vi "battery-reader-dialog.vi"() -> ()   [LabVIEW 2025]
uses:
  <vilib>/addons/_JKI Toolkits/State Machine/_JKI_lib_State_Machine.llb/Select State(s)_err__jki_lib_state_machine.vi
  <vilib>/addons/_JKI Toolkits/State Machine/_JKI_lib_State_Machine.llb/Periodic Trigger__ogtk__JKI-SM__jki_lib_state_machine.vi
  artifacts/battery-prompt/battery-prompt.lvlibp
panel:
  out "DONE":bool
  out "Battery data":T1
  out "Raw content":string
  in  "Restart":bool
  in  "Send request":bool
  in  "Read image":bool
  in  "Exit":bool
  in  "Image selection":enum32{"Camera", "File input"}(tab)
  out "Acquired picture":picture
  in  "Pict Ring":u16(ring)
  out "error out":errorcluster
  in  "error in":errorcluster
  in  "Camera ID":u8
  # "AI-Powered Battery Testing: Prototype Integration of LabVIEW and OpenAI"
  # "1. Select the camera ID and read the image."
  # "2. Use camera input, or select one of the predefined templates."
  # "3. Inspect the data received from the GPT"
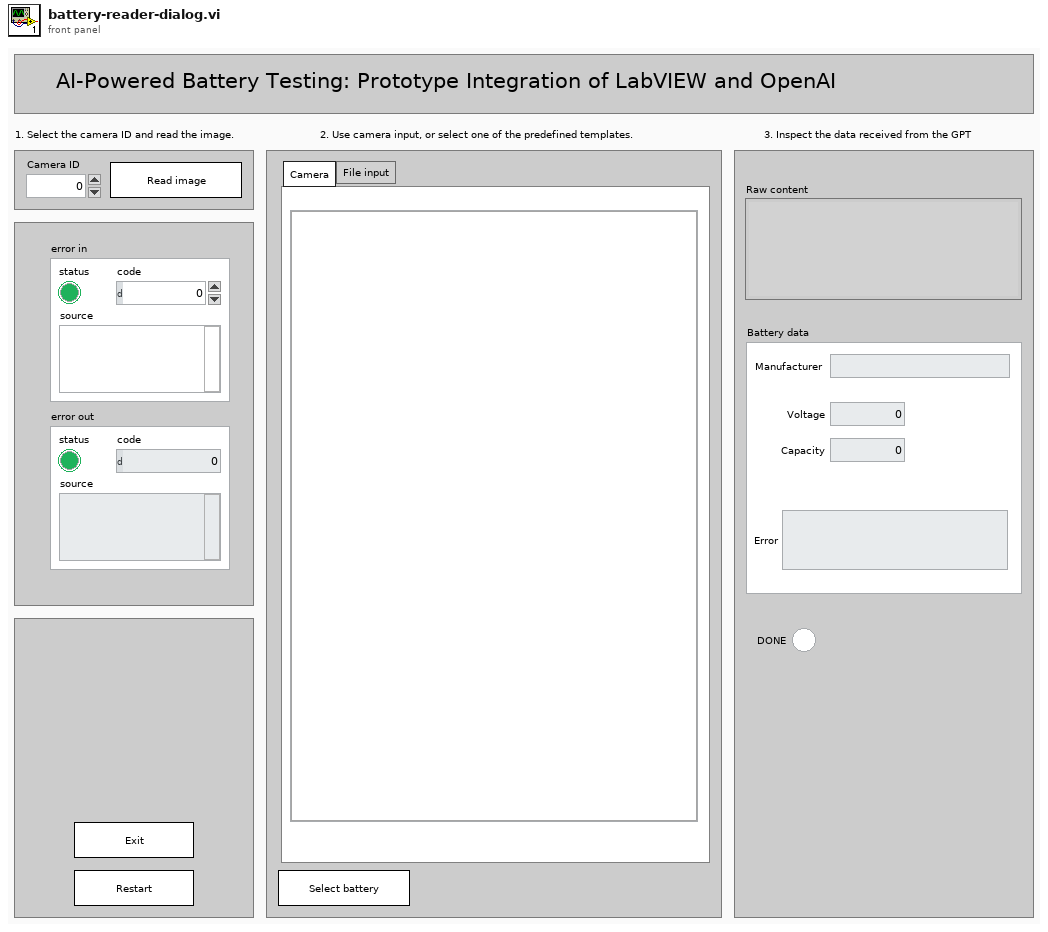
[diagram p1: front panel]
types:
  T1 = cluster{"Manufacturer":string, "Voltage":dbl, "Capacity":u32, "Error":string}
  T2 = enum32{"Invalid", "Standard", "Closed", "Hidden", "Minimized", "Maximized"}
  T3 = enum32{"invalid app kind", "Development System", "Run Time System", "Student Edition", "Embedded LabVIEW", "Evaluation", "Custom"}
  T4 = enum8{"Enabled", "Disabled", "Disabled and Grayed Out"}
  T5 = cluster{"Core":cluster{"Current VI Reference":refnum<vi>, "Close Panel on Exit?":bool}, "Camera ID":u8, "Acquired image":path}
  T6 = cluster{"Current VI Reference":refnum<vi>, "Close Panel on Exit?":bool}
  T7 = typedef "imagedata.ctl" = cluster{"image type":i32, "image depth":i32, "image":u8[], "mask":u8[], "colors":u32[], "Rectangle":cluster{"left":i16, "top":i16, "right":i16, "bottom":i16}}
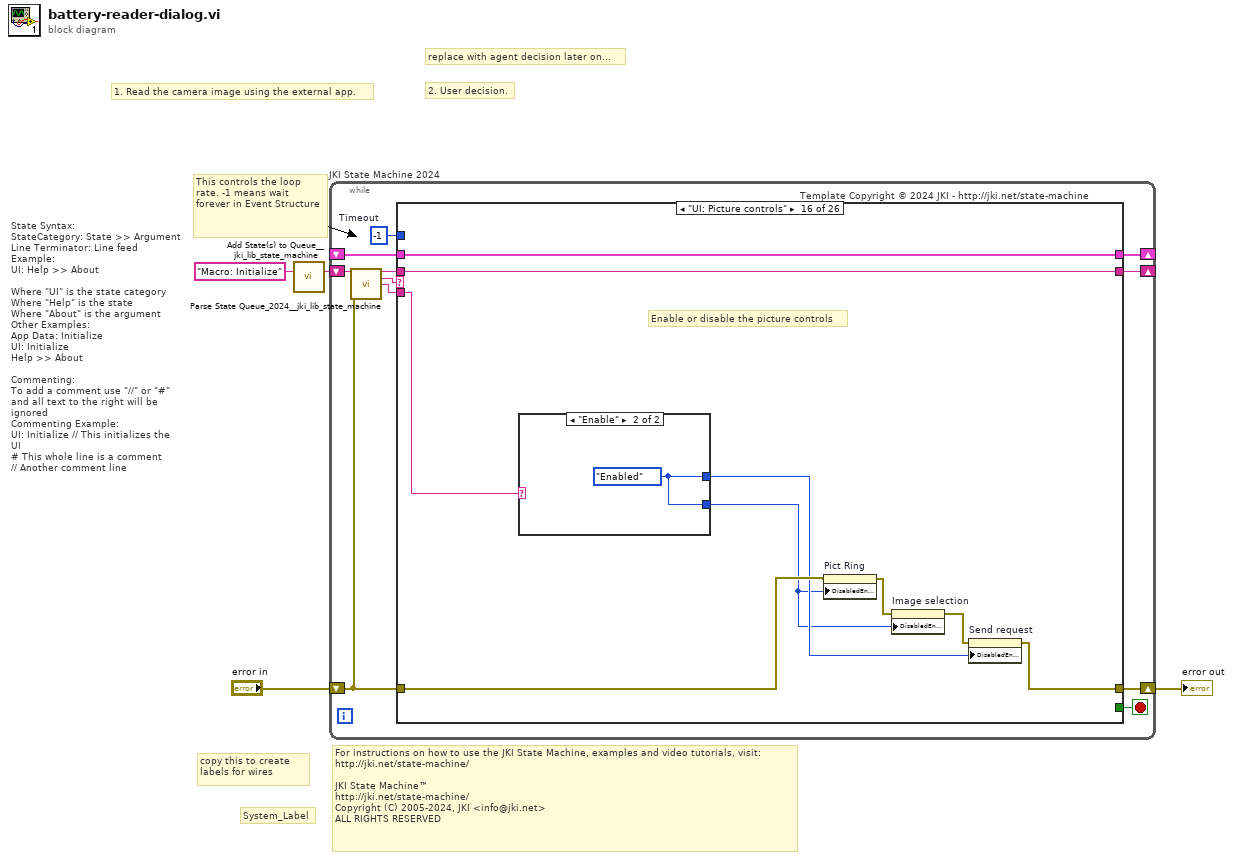
[diagram p0: block diagram]
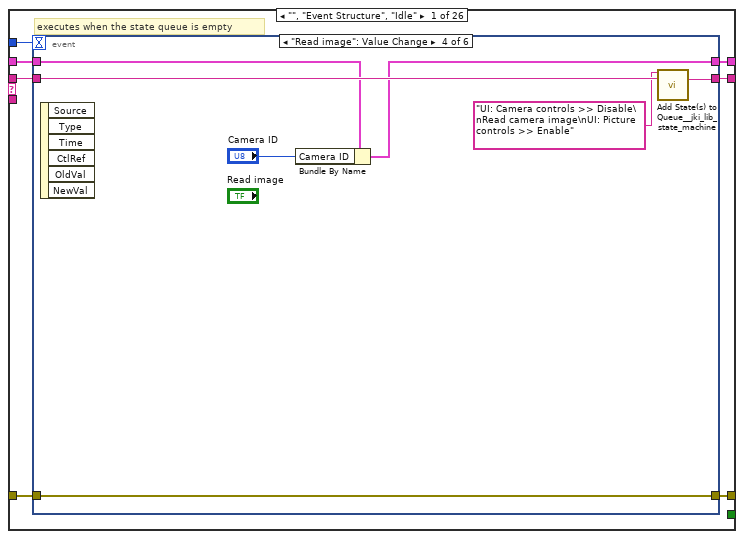
[diagram p2: hidden frame]
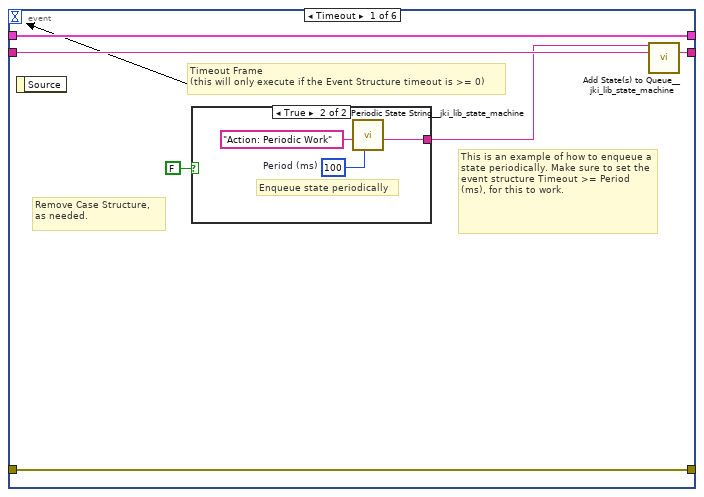
[diagram p3: hidden frame]
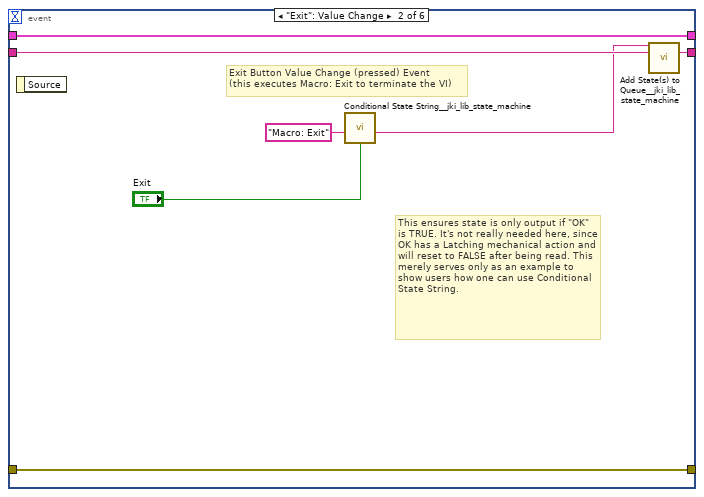
[diagram p5: hidden frame]
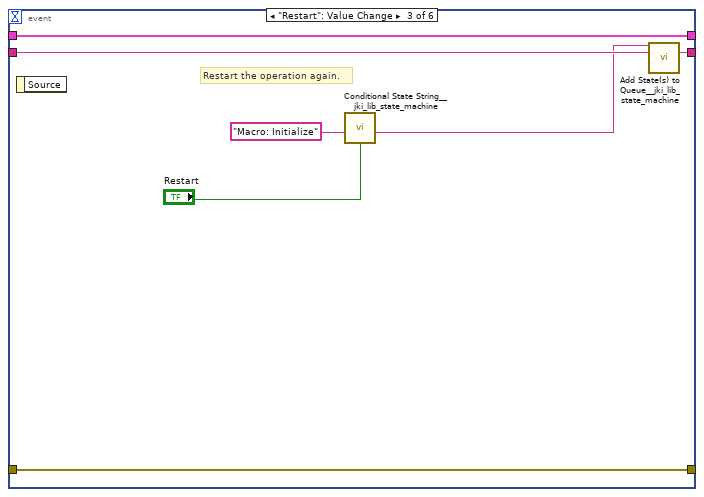
[diagram p6: hidden frame]
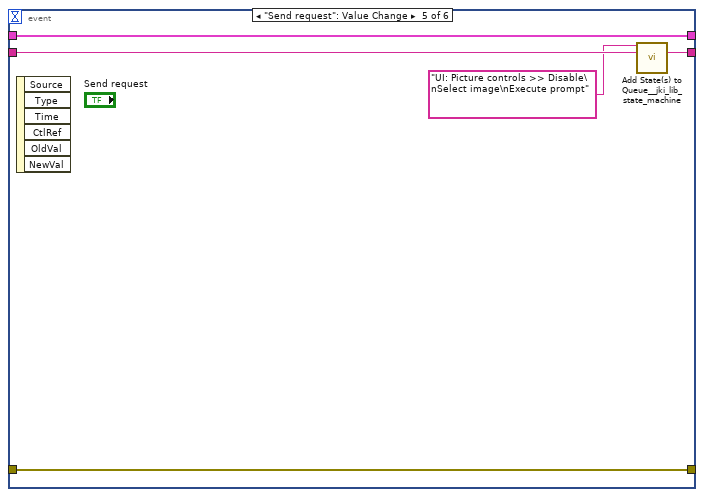
[diagram p7: hidden frame]
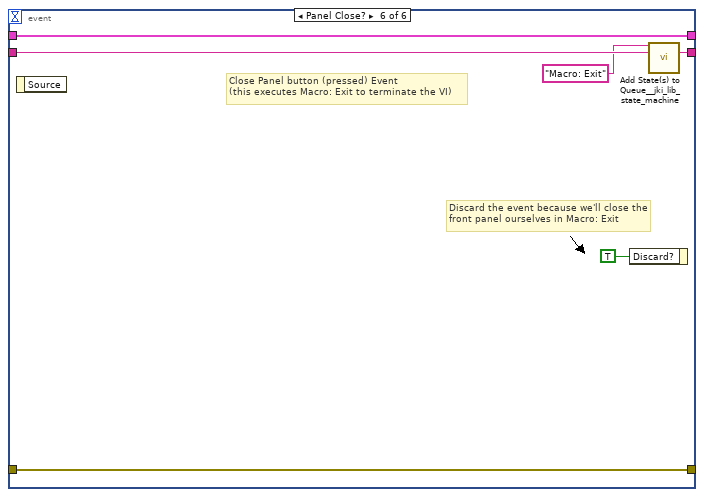
[diagram p8: hidden frame]
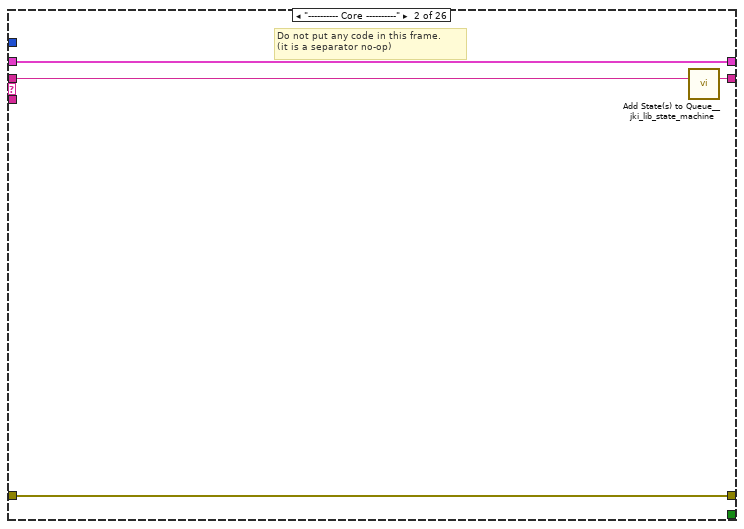
[diagram p9: hidden frame]
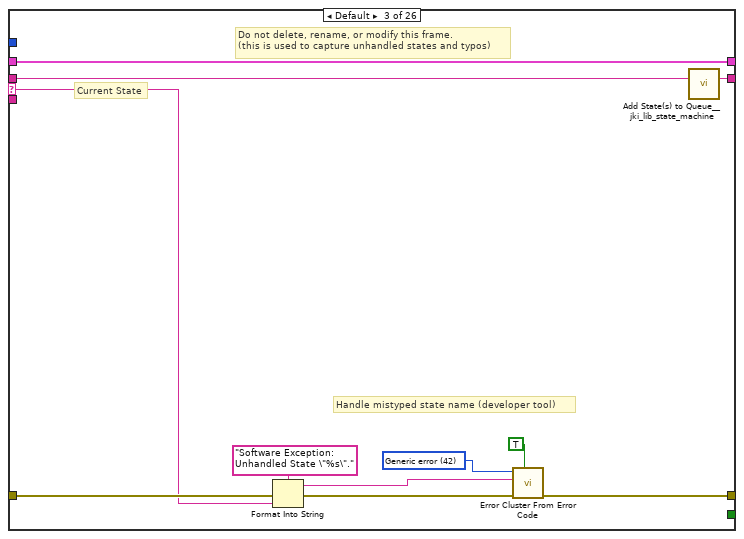
[diagram p10: hidden frame]
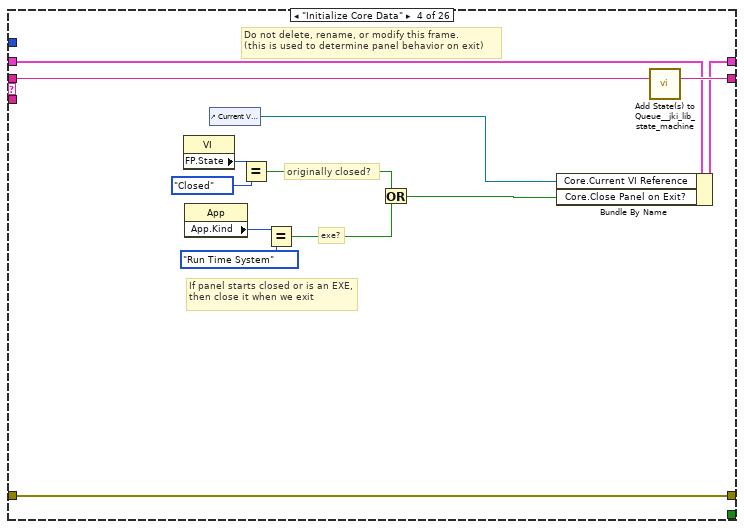
[diagram p11: hidden frame]
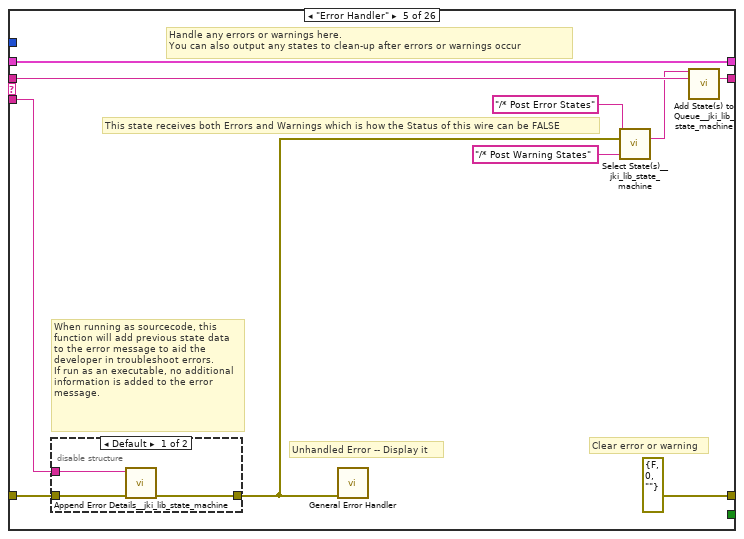
[diagram p12: hidden frame]
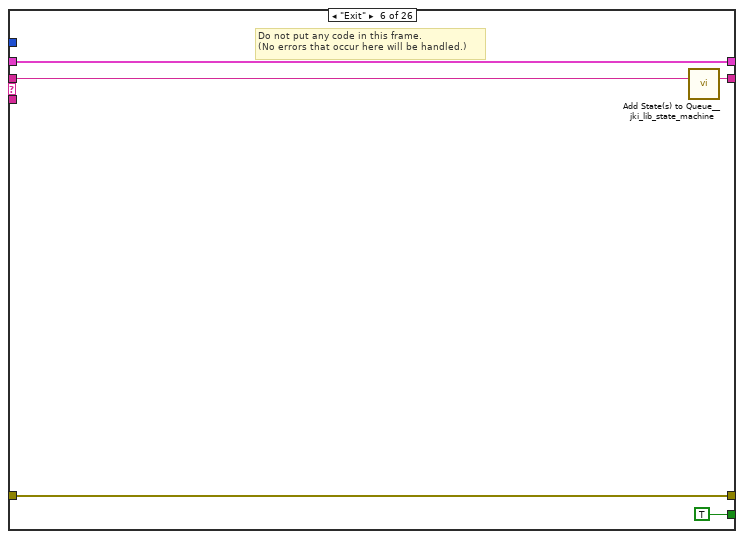
[diagram p14: hidden frame]
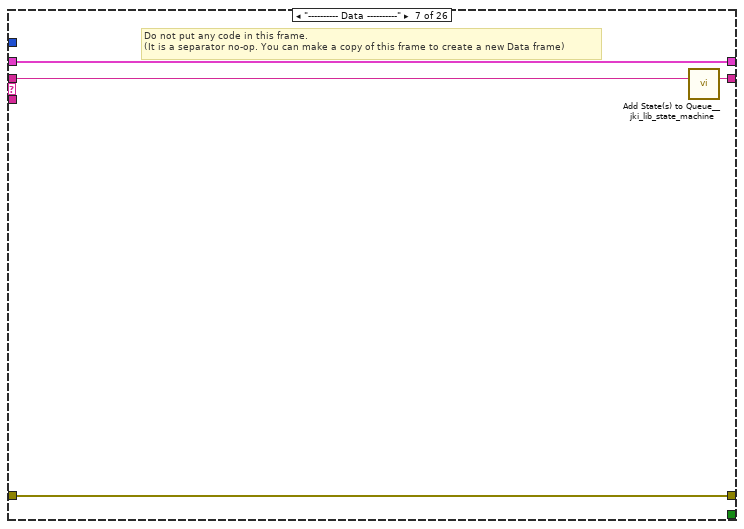
[diagram p15: hidden frame]
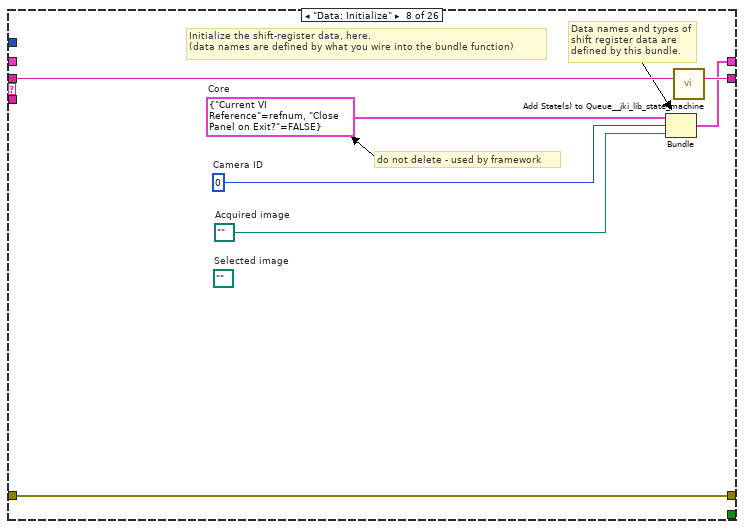
[diagram p16: hidden frame]
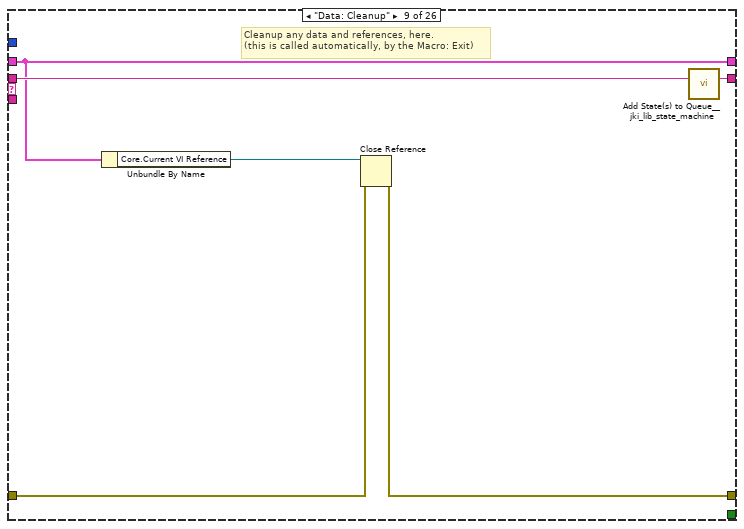
[diagram p17: hidden frame]
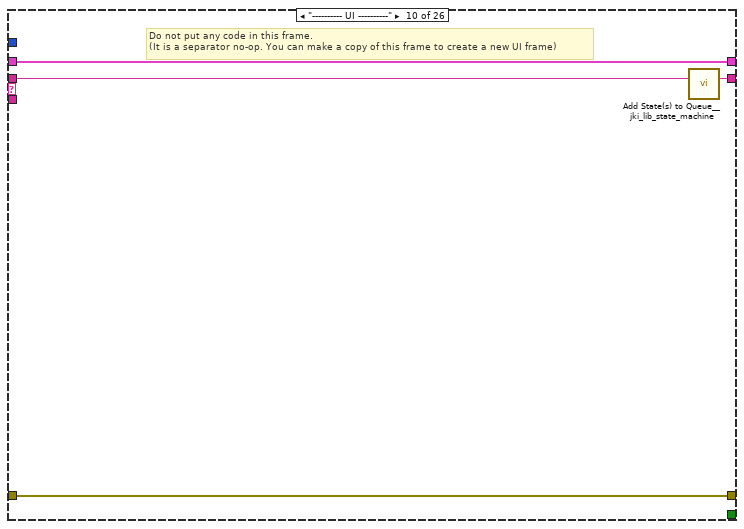
[diagram p18: hidden frame]
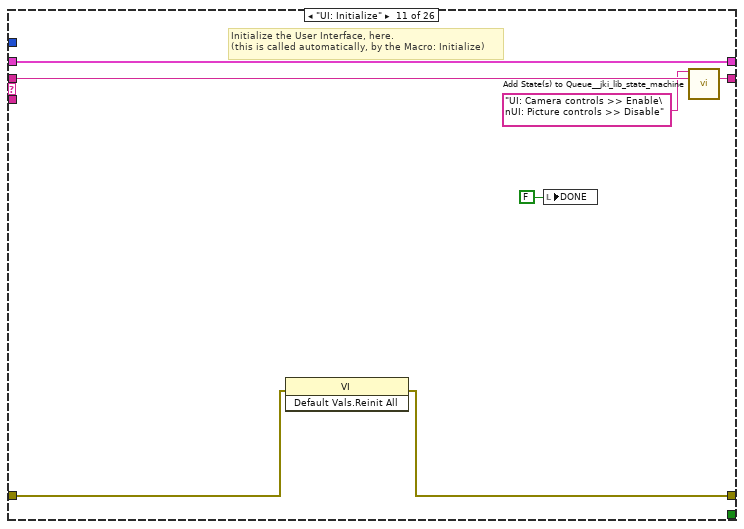
[diagram p19: hidden frame]
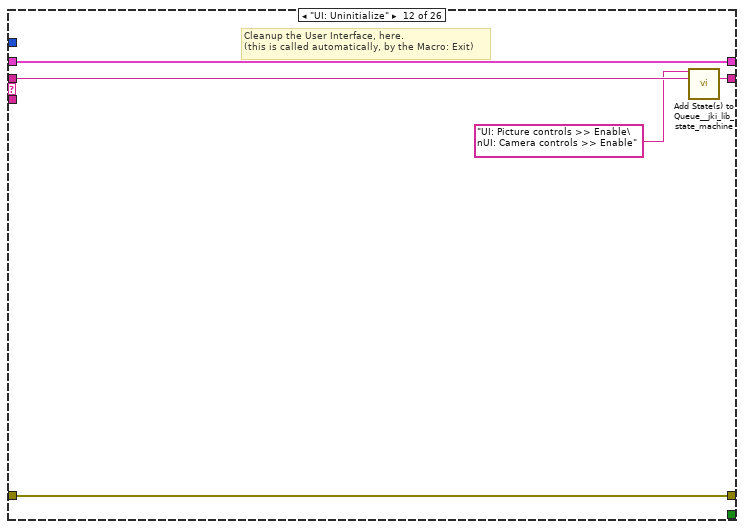
[diagram p20: hidden frame]
diagram:
  # "For instructions on how to use the JKI State Machine, examples and video tutorials, visit:\nhttp://jki.net/state-machine/\n\nJKI State Machine™\nhttp://jki.net/state-machine/\nCopyright (C) 2005-2024, JKI <info@jki.net>\nALL RIGHTS RESERVED"
  # "State Syntax:\nStateCategory: State >> Argument\nLine Terminator: Line feed\nExample:\nUI: Help >> About\n\nWhere \"UI\" is the state category\nWhere \"Help\" is the state\nWhere \"About\" is the argument\nOther Examples:\nApp Data: Initialize\nUI: Initialize\nHelp >> About\n\nCommenting:\nTo add a comment use \"//\" or \"#\" and all text to the right will be ignored\nCommenting Example:\nUI: Initialize // This initializes the UI\n# This whole line is a comment\n// Another comment line"
  # "copy this to create labels for wires"
  # "This controls the loop rate. -1 means wait forever in Event Structure"
  # "System_Label"
  # "replace with agent decision later on..."
  # "2. User decision."
  # "1. Read the camera image using the external app."
  n1 = call <vilib>:"Add State(s) to Queue__jki_lib_state_machine.vi"("State(s) in (\"\")"="Macro: Initialize") -> ("States Out"=w4:string)  [unwired: 14 in]
  n2 = while "JKI State Machine 2024" {
    shift-right: [w8] -> _
    shift-left: _ -> [w7]
    shift-right: [w11] -> w2
    shift-left: "error in" -> [w5]
    shift-right: [w10] -> _
    shift-left: w4 -> [w12]
    stop <- w9 stop-if-true
    w6 = -1  # Timeout
    # "Template Copyright © 2024 JKI - http://jki.net/state-machine"
    n3 = call <vilib>:"Parse State Queue_2024__jki_lib_state_machine.vi"("State Queue"=w12, "Error In (no error)"=w5) -> ("Remaining States"=w14:string, "Current State"=w15:string, "Arguments"=w13:string)  [unwired: 11 in]
    n4 = case shown="\"UI: Picture controls\"" w15 {
      selector: w15 -> [_ _ w68 _ _ _ _ _ _ _ _ _ _ _ _ _ _ _ _ _ _ _ _ _ _ _]
      tunnel: w14 -> [w22 w67 w72 w91 w101 w110 w114 w121 w127 w131 w138 w143 w149 w160 w231 w242 w250 w255 w264 w268 w272 w276 w291 w300 w313 w340]
      tunnel: w13 -> [_ _ _ _ w96 _ _ _ _ _ _ _ w144 w154 w229 w241 _ _ _ _ _ _ _ _ _ w338]
      tunnel: w7 -> [w20 w64 w70 w84 w98 w108 w111 _ w122 w128 w136 w141 w147 w156 w232 w243 w247 w252 w262 w265 w269 w273 w283 w293 w331 w341]
      tunnel: [w19 w65 w74 w88 errorcluster {"status"=FALSE, "code"=0, "source"=""} ("error out") w107 w112 w118 w123 w129 w132 w140 w145 w157 w227 w237 w248 w253 w259 w266 w270 w274 w278 w299 w320 w333] -> w11
      tunnel: w5 -> [w16 w65 w73 w88 w97 w107 w112 w118 w124 w129 w133 w140 w146 w158 w230 w240 w248 w253 w259 w266 w270 w274 w290 w299 w330 w339]
      tunnel: [w21 w66 w71 w90 w100 w109 w113 w120 w126 w130 w137 w142 w148 w159 w231 w242 w249 w254 w263 w267 w271 w275 w291 w300 w314 w340] -> w10
      tunnel: [_ _ _ _ _ TRUE _ _ _ _ _ _ _ _ _ _ _ _ _ _ _ _ _ _ _ _] -> w9
      tunnel: [w18 w64 w70 w89 w98 w108 w111 w119 w122 w128 w136 w141 w147 w156 w232 w243 w247 w252 w262 w265 w269 w273 w282 w292 w331 w341] -> w8
      tunnel: w6 -> [w17 _ _ _ _ _ _ _ _ _ _ _ _ _ _ _ _ _ _ _ _ _ _ _ _ _]
      frame "", "Event Structure", "Idle" {
        # "executes when the state queue is empty"
        n5 = event shown="[3] \"Read image\": Value Change" {
          selector: _ -> [_ _ _ _ _ _]
          dyn-events: _ -> [_ _ _ _ _ _]
          timeout: w17 -> [_ _ _ _ _ _]
          tunnel: w22 -> [w28 w38 w45 w52 w55 w63]
          tunnel: [w27 w37 w44 w51 w56 w62] -> w21
          tunnel: w20 -> [w25 w35 w42 w48 w57 w60]
          tunnel: [w26 w36 w43 w49 w53 w61] -> w19
          tunnel: w16 -> [w26 w36 w43 w49 w53 w61]
          tunnel: [w25 w35 w42 w46 w57 w60] -> w18
          event Timeout {
            # "Remove Case Structure, as needed."
            # "This is an example of how to enqueue a state periodically. Make sure to set the event structure Timeout >= Period (ms), for this to work."
            # "Timeout Frame\n(this will only execute if the Event Structure timeout is >= 0)"
            n6 = event-data() -> ()  [unwired: 1 in, 1 out]
            n7 = case shown="True" FALSE {
              tunnel: [_ w31] -> w24
              frame False {
              }
              frame True {
                w29 = u32 100  # Period (ms)
                # "Enqueue state periodically"
                n8 = call <vilib>:"Periodic State String__jki_lib_state_machine.vi"("Period (ms)"=w29, "State"="Action: Periodic Work") -> ("State Out"=w31:string)  [unwired: 9 in]
              }
            }
            n9 = call <vilib>:"Add State(s) to Queue__jki_lib_state_machine.vi"("State(s) in Front (\"\")"=w24, "State(s) in (\"\")"=w28) -> ("States Out"=w27:string)  [unwired: 13 in]
          }
          event "Exit": Value Change {
            # "This ensures state is only output if \"OK\" is TRUE. It's not really needed here, since OK has a Latching mechanical action and will reset to FALSE after being read. This merely serves only as an example to show users how one can use Conditional State String."
            # "Exit Button Value Change (pressed) Event\n(this executes Macro: Exit to terminate the VI)"
            n10 = event-data() -> ()  [unwired: 1 in, 1 out]
            n11 = call <vilib>:"Conditional State String__jki_lib_state_machine.vi"("Do State(s)?"="Exit", "State"="Macro: Exit") -> ("State Out"=w32:string)  [unwired: 7 in]
            n12 = call <vilib>:"Add State(s) to Queue__jki_lib_state_machine.vi"("State(s) in Front (\"\")"=w32, "State(s) in (\"\")"=w38) -> ("States Out"=w37:string)  [unwired: 13 in]
          }
          event "Restart": Value Change {
            # "Restart the operation again."
            n13 = event-data() -> ()  [unwired: 1 in, 1 out]
            n14 = call <vilib>:"Conditional State String__jki_lib_state_machine.vi"("Do State(s)?"="Restart", "State"="Macro: Initialize") -> ("State Out"=w40:string)  [unwired: 7 in]
            n15 = call <vilib>:"Add State(s) to Queue__jki_lib_state_machine.vi"("State(s) in Front (\"\")"=w40, "State(s) in (\"\")"=w45) -> ("States Out"=w44:string)  [unwired: 13 in]
          }
          event "Read image": Value Change {
            n16 = event-data() -> ()  [unwired: 1 in, 6 out]
            n17 = Bundle By Name(cluster=w48, "Camera ID"="Camera ID") -> (w46:T5)
            n18 = call <vilib>:"Add State(s) to Queue__jki_lib_state_machine.vi"("State(s) in Front (\"\")"="UI: Camera controls >> Disable\nRead camera image\nUI: Picture controls >> Enable" ("State(s) in Front (\"\")"), "State(s) in (\"\")"=w52) -> ("States Out"=w51:string)  [unwired: 13 in]
          }
          event "Send request": Value Change {
            n19 = event-data() -> ()  [unwired: 1 in, 6 out]
            n20 = call <vilib>:"Add State(s) to Queue__jki_lib_state_machine.vi"("State(s) in Front (\"\")"="UI: Picture controls >> Disable\nSelect image\nExecute prompt" ("State(s) in Front (\"\")"), "State(s) in (\"\")"=w55) -> ("States Out"=w56:string)  [unwired: 13 in]
          }
          event Panel Close? {
            # "Discard the event because we'll close the front panel ourselves in Macro: Exit"
            # "Close Panel button (pressed) Event\n(this executes Macro: Exit to terminate the VI)"
            n21 = event-data() -> ()  [unwired: 1 in, 1 out]
            n22 = event-data("Discard?"=TRUE) -> ()  [unwired: 1 in, 1 out]
            n23 = call <vilib>:"Add State(s) to Queue__jki_lib_state_machine.vi"("State(s) in Front (\"\")"="Macro: Exit", "State(s) in (\"\")"=w63) -> ("States Out"=w62:string)  [unwired: 13 in]
          }
        }
      }
      frame "---------- Core ----------" {
        # "Do not put any code in this frame.\n(it is a separator no-op)"
        n24 = call <vilib>:"Add State(s) to Queue__jki_lib_state_machine.vi"("State(s) in (\"\")"=w67) -> ("States Out"=w66:string)  [unwired: 14 in]
      }
      frame Default {
        w77 = 42 items=["No error", "Argument error", "Memory is full", "Out of zone", "End of file", "File already open", "Generic file I/O error", "File not found", "File permission error", "Disk is full", "Duplicate path", "Too many files open", "System feature not enabled", "Resource file not found", "Cannot add resource", "Resource not found", "Image not found", "Image memory error", "Pen does not exist", "Config type invalid", "Config token not found", "Config parse error", "Config memory error", "Bad external code format", "Bad external code offset", "External code not present", "Null window", "Destroy window error", "Null menu", "Print aborted", "Bad print record", "Print driver error", "Windows error during printing", "Memory error during printing", "Print dialog error", "Generic print error", "Invalid device refnum", "Device not found", "Device parameter error", "Device unit error", "Cannot open device", "Device call aborted", "Generic error", "Cancelled by user", "Object ID too low", "Object ID too high", "Object not in heap", "Unknown heap", "Unknown object (invalid DefProc)", "Unknown object (DefProc not in table)", "Message out of range", "Invalid (null) method", "Unknown message", "Manager call not supported", "Bad address", "Network operation in progress", "Network operation timed out", "Connection is busy", "Network attribute not supported", "Network error", "Address in use", "System out of memory", "Connection aborted", "Connection refused", "Not connected", "Already connected", "Connection closed", "Initialization error (interapplication manager)", "Bad occurrence", "Wait on unbound occurrence handler", "Occurrence queue overflow", "Datalog type conflict", "Unused", "Unrecognized type (interapplication manager)", "Memory corrupt", "Failed to make temporary DLL", "Old CIN version", "Drag socket not found", "Failed to load drop-object", "Failed to register OLE object", "Failed to release OLE object", "Format specifier type mismatch", "Unknown format specifier", "Too few format specifiers", "Too many format specifiers", "Scan failed", "Newer CIN version", "Error converting to variant", "Runtime menu error", "Password tampered", "Variant attribute not found", "Incompatible variant data type", "Event data is not available", "Event Store is not present", "Occurrence is not found", "Event Queue is not created", "Event info is not available", "Refnum passed is NULL", "Error retrieving Class GUID", "Error retrieving CoClass GUID", "Error retrieving TypeLib GUID.", "Bad built application magic bytes.", "Specific driver is different from the specific driver associated with the Logical Name.", "There is no session opened to the class driver.", "Max Error", "MAX - Error with config objects", "MAX - Error loading configuration", "MAX - Group not supported"]
        # "Current State"
        # "Do not delete, rename, or modify this frame.\n(this is used to capture unhandled states and typos)"
        # "Handle mistyped state name (developer tool)"
        n25 = Format Into String(format string="Software Exception: Unhandled State \"%s\"." ("message"), error in=w73, w68) -> (resulting string=w76:string, error out=w75:errorcluster)  [unwired: 1 in]
        n26 = call <vilib>:"Error Cluster From Error Code.vi"("show call chain? (False)"=TRUE, "error in (no error)"=w75, "error message (\"\")"=w76, "error code (0)"=w77) -> ("error out"=w74:errorcluster)  [unwired: 5 in]
        n27 = call <vilib>:"Add State(s) to Queue__jki_lib_state_machine.vi"("State(s) in (\"\")"=w72) -> ("States Out"=w71:string)  [unwired: 14 in]
      }
      frame "Initialize Core Data" {
        # "Do not delete, rename, or modify this frame.\n(this is used to determine panel behavior on exit)"
        # "originally closed?"
        # "exe?"
        # "If panel starts closed or is an EXE, then close it when we exit"
        n28 = property class="VI"() -> ("FP.State"=w81:T2)  [unwired: 2 in, 2 out]
        n29 = property class="App"() -> ("App.Kind"=w87:T3)  [unwired: 2 in, 2 out]
        n30 = control-ref of="Current VI Reference"() -> (w82:refnum<vi>)
        n31 = Equal?(x=w81, y=T2."Closed" ("Front Panel Window:State")) -> (x = y?=w79:bool)
        n32 = Equal?(x=w87, y=T3."Run Time System" ("Application:Kind")) -> (x = y?=w85:bool)
        n33 = Or(x=w79, y=w85) -> (x .or. y?=w83:bool)
        n34 = Bundle By Name(cluster=w84, "Core.Current VI Reference"=w82, "Core.Close Panel on Exit?"=w83) -> (w89:T5)
        n35 = call <vilib>:"Add State(s) to Queue__jki_lib_state_machine.vi"("State(s) in (\"\")"=w91) -> ("States Out"=w90:string)  [unwired: 14 in]
      }
      frame "Error Handler" {
        # "When running as sourcecode, this function will add previous state data to the error message to aid the developer in troubleshoot errors.\nIf run as an executable, no additional information is added to the error message."
        # "This state receives both Errors and Warnings which is how the Status of this wire can be FALSE"
        # "Unhandled Error -- Display it"
        # "Handle any errors or warnings here.\nYou can also output any states to clean-up after errors or warnings occur"
        # "Clear error or warning"
        n36 = disable-structure shown="Default" {
          disable-tunnel: w97 -> [w104 w105]
          disable-tunnel: w96 -> [w103 _]
          disable-tunnel: [w102 w105] -> w95
          frame condition #0 (active) {
            n37 = call <vilib>:"Append Error Details__jki_lib_state_machine.vi"("error in (no error)"=w104, "Previous State and Argument(s)"=w103) -> ("error out"=w102:errorcluster)  [unwired: 9 in]
          }
          frame condition #1 {
          }
        }
        n38 = call <vilib>:"General Error Handler.vi"("error in (no error)"=w95) -> ()  [unwired: 10 in, 5 out]
        n39 = call-poly <vilib>:"Select State(s)__jki_lib_state_machine.vi"("State(s) if True (\"\")"="/* Post Error States", "Select"=w95, "State(s) if False (\"\")"="/* Post Warning States") -> ("States Out"=w93:string)  [unwired: 12 in]
        n40 = call <vilib>:"Add State(s) to Queue__jki_lib_state_machine.vi"("State(s) in Front (\"\")"=w93, "State(s) in (\"\")"=w101) -> ("States Out"=w100:string)  [unwired: 13 in]
      }
      frame "Exit" {
        # "Do not put any code in this frame.\n(No errors that occur here will be handled.)"
        n41 = call <vilib>:"Add State(s) to Queue__jki_lib_state_machine.vi"("State(s) in (\"\")"=w110) -> ("States Out"=w109:string)  [unwired: 14 in]
      }
      frame "---------- Data ----------" {
        # "Do not put any code in this frame.\n(It is a separator no-op. You can make a copy of this frame to create a new Data frame)"
        n42 = call <vilib>:"Add State(s) to Queue__jki_lib_state_machine.vi"("State(s) in (\"\")"=w114) -> ("States Out"=w113:string)  [unwired: 14 in]
      }
      frame "Data: Initialize" {
        (unwired) path ""  # Selected image
        w115 = path ""  # Acquired image
        w116 = u8 0  # Camera ID
        w117 = T6 {"Current VI Reference"=refnum, "Close Panel on Exit?"=FALSE}  # Core
        # "do not delete - used by framework"
        # "Data names and types of shift register data are defined by this bundle."
        # "Initialize the shift-register data, here.\n(data names are defined by what you wire into the bundle function)"
        n43 = Bundle("Core"=w117, "Camera ID"=w116, "Acquired image"=w115) -> (w119:T5)  [unwired: 1 in]
        n44 = call <vilib>:"Add State(s) to Queue__jki_lib_state_machine.vi"("State(s) in (\"\")"=w121) -> ("States Out"=w120:string)  [unwired: 14 in]
      }
      frame "Data: Cleanup" {
        # "Cleanup any data and references, here.\n(this is called automatically, by the Macro: Exit)"
        n45 = Unbundle By Name(w122) -> ("Core.Current VI Reference"=w125:refnum<vi>)
        n46 = Close Reference(reference=w125, error in (no error)=w124) -> (error out=w123:errorcluster)
        n47 = call <vilib>:"Add State(s) to Queue__jki_lib_state_machine.vi"("State(s) in (\"\")"=w127) -> ("States Out"=w126:string)  [unwired: 14 in]
      }
      frame "---------- UI ----------" {
        # "Do not put any code in this frame.\n(It is a separator no-op. You can make a copy of this frame to create a new UI frame)"
        n48 = call <vilib>:"Add State(s) to Queue__jki_lib_state_machine.vi"("State(s) in (\"\")"=w131) -> ("States Out"=w130:string)  [unwired: 14 in]
      }
      frame "UI: Initialize" {
        # "Initialize the User Interface, here.\n(this is called automatically, by the Macro: Initialize)"
        n49 = invoke class="VI" method="Default Vals.Reinit All"(error in=w133) -> (error out=w132:errorcluster)  [unwired: 2 in, 2 out]
        n50 = local write "DONE"(FALSE ("DONE")) -> ()
        n51 = call <vilib>:"Add State(s) to Queue__jki_lib_state_machine.vi"("State(s) in Front (\"\")"="UI: Camera controls >> Enable\nUI: Picture controls >> Disable" ("State(s) in Front (\"\")"), "State(s) in (\"\")"=w138) -> ("States Out"=w137:string)  [unwired: 13 in]
      }
      frame "UI: Uninitialize" {
        # "Cleanup the User Interface, here.\n(this is called automatically, by the Macro: Exit)"
        n52 = call <vilib>:"Add State(s) to Queue__jki_lib_state_machine.vi"("State(s) in Front (\"\")"="UI: Picture controls >> Enable\nUI: Camera controls >> Enable" ("State(s) in Front (\"\")"), "State(s) in (\"\")"=w143) -> ("States Out"=w142:string)  [unwired: 13 in]
      }
      frame "UI: Cursor Set" {
        # "Argument"
        # "Set and Unset Cursor Busy.\n(Usage: \"UI: Cursor Set >> Busy|Idle\")"
        n53 = case shown="\"Idle\", Default" w144 {
          tunnel: w146 -> [w151 w153]
          tunnel: [w150 w152] -> w145
          frame "Idle", Default {
            n54 = call <vilib>:"Unset Busy.vi"("error in (no error)"=w151) -> ("error out"=w150:errorcluster)  [unwired: 10 in]
          }
          frame "Busy" {
            n55 = call <vilib>:"Set Busy.vi"("error in (no error)"=w153) -> ("error out"=w152:errorcluster)  [unwired: 9 in, 1 out]
          }
        }
        n56 = call <vilib>:"Add State(s) to Queue__jki_lib_state_machine.vi"("State(s) in (\"\")"=w149) -> ("States Out"=w148:string)  [unwired: 14 in]
      }
      frame "UI: Front Panel State" {
        # "Argument"
        # "Set Front Panel Open or Closed\n(Usage: \"UI: Front Panel State >> Open|Close\")"
        n57 = Unbundle By Name(w156) -> ("Core.Current VI Reference"=w155:refnum<vi>)
        n58 = case shown="\"Close\", \"Closed\"" w154 {
          tunnel: w158 -> [w166 w181 w192 w205 w218]
          tunnel: [w168 w182 w194 w207 w220] -> w157
          tunnel: w155 -> [w167 w179 w193 w206 w219]
          frame "Open", "Standard", Default {
            w161 = T2."Standard" ("State")
            n59 = property class="VI"(reference=w167, error in=w166) -> (reference out=w164:refnum<vi>, error out=w165:errorcluster, "FP.State"=w163:T2)
            n60 = Not Equal?(x=w163, y=w161) -> (x != y?=w162:bool)
            n61 = case shown="True" w162 {
              tunnel: [w172 w174] -> w168
              tunnel: w165 -> [w171 w174]
              tunnel: w164 -> [w170 _]
              tunnel: w161 -> [w169 _]
              frame True {
                n62 = invoke class="VI" method="FP.Open"(reference=w170, error in=w171, "Activate"=TRUE, "State"=w169) -> (error out=w172:errorcluster)  [unwired: 1 in, 4 out]
              }
              frame False {
              }
            }
          }
          frame "Close", "Closed" {
            n63 = property class="VI"(reference=w179, error in=w181) -> (reference out=w178:refnum<vi>, error out=w180:errorcluster, "FP.State"=w176:T2)
            n64 = Not Equal?(x=w176, y=T2."Closed" ("Front Panel Window:State")) -> (x != y?=w175:bool)
            n65 = case shown="True" w175 {
              tunnel: [w183 w186] -> w182
              tunnel: w180 -> [w183 w185]
              tunnel: w178 -> [_ w184]
              frame False {
              }
              frame True {
                n66 = invoke class="VI" method="FP.Close"(reference=w184, error in=w185) -> (error out=w186:errorcluster)  [unwired: 1 in, 2 out]
              }
            }
          }
          frame "Hidden", "Hide" {
            w187 = T2."Hidden" ("State")
            n67 = property class="VI"(reference=w193, error in=w192) -> (reference out=w190:refnum<vi>, error out=w191:errorcluster, "FP.State"=w189:T2)
            n68 = Not Equal?(x=w189, y=w187) -> (x != y?=w188:bool)
            n69 = case shown="True" w188 {
              tunnel: [w198 w199] -> w194
              tunnel: w191 -> [w197 w199]
              tunnel: w190 -> [w196 _]
              tunnel: w187 -> [w195 _]
              frame True {
                n70 = invoke class="VI" method="FP.Open"(reference=w196, error in=w197, "State"=w195) -> (error out=w198:errorcluster)  [unwired: 2 in, 4 out]
              }
              frame False {
              }
            }
          }
          frame "Minimize", "Minimized" {
            w200 = T2."Minimized" ("State")
            n71 = property class="VI"(reference=w206, error in=w205) -> (reference out=w203:refnum<vi>, error out=w204:errorcluster, "FP.State"=w202:T2)
            n72 = Not Equal?(x=w202, y=w200) -> (x != y?=w201:bool)
            n73 = case shown="True" w201 {
              tunnel: [w211 w212] -> w207
              tunnel: w204 -> [w210 w212]
              tunnel: w203 -> [w209 _]
              tunnel: w200 -> [w208 _]
              frame True {
                n74 = invoke class="VI" method="FP.Open"(reference=w209, error in=w210, "State"=w208) -> (error out=w211:errorcluster)  [unwired: 2 in, 4 out]
              }
              frame False {
              }
            }
          }
          frame "Maximize", "Maximized" {
            w213 = T2."Maximized" ("State")
            n75 = property class="VI"(reference=w219, error in=w218) -> (reference out=w216:refnum<vi>, error out=w217:errorcluster, "FP.State"=w215:T2)
            n76 = Not Equal?(x=w215, y=w213) -> (x != y?=w214:bool)
            n77 = case shown="True" w214 {
              tunnel: [w224 w225] -> w220
              tunnel: w217 -> [w223 w225]
              tunnel: w216 -> [w222 _]
              tunnel: w213 -> [w221 _]
              frame True {
                n78 = invoke class="VI" method="FP.Open"(reference=w222, error in=w223, "State"=w221) -> (error out=w224:errorcluster)  [unwired: 2 in, 4 out]
              }
              frame False {
              }
            }
          }
        }
        n79 = call <vilib>:"Add State(s) to Queue__jki_lib_state_machine.vi"("State(s) in (\"\")"=w160) -> ("States Out"=w159:string)  [unwired: 14 in]
      }
      frame "UI: Camera controls" {
        # "Enable or disable the camera controls"
        n80 = case shown="\"Enable\"" w229 {
          tunnel: [T4."Disabled and Grayed Out" ("Disabled") T4."Enabled" ("Disabled")] -> w226
          frame "Disable", Default {
          }
          frame "Enable" {
          }
        }
        n81 = property on="Camera ID" class="DigNum (strict)"(error in=w230, "DisabledEnum"=w226) -> (error out=w228:errorcluster)  [unwired: 1 in, 1 out]
        n82 = property on="Read image" class="Bool"(error in=w228, "DisabledEnum"=w226) -> (error out=w227:errorcluster)  [unwired: 1 in, 1 out]
      }
      frame "UI: Picture controls" {
        # "Enable or disable the picture controls"
        n83 = case shown="\"Enable\"" w241 {
          tunnel: [T4."Disabled and Grayed Out" ("Disabled") w246] -> w236
          tunnel: [T4."Disabled" ("Disabled") w246] -> w235
          frame "Disable", Default {
          }
          frame "Enable" {
            w246 = T4."Enabled" ("Disabled")
          }
        }
        n84 = property on="Pict Ring" class="Ring (strict)"(error in=w240, "DisabledEnum"=w235) -> (error out=w239:errorcluster)  [unwired: 1 in, 1 out]
        n85 = property on="Image selection" class="TabCtl (strict)"(error in=w239, "DisabledEnum"=w235) -> (error out=w238:errorcluster)  [unwired: 1 in, 1 out]
        n86 = property on="Send request" class="Bool"(error in=w238, "DisabledEnum"=w236) -> (error out=w237:errorcluster)  [unwired: 1 in, 1 out]
      }
      frame "---------- Macro ----------" {
        # "Do not put any code in this frame.\n(It is a separator no-op. You can make a copy of this frame to create a new Macro frame)"
        n87 = call <vilib>:"Add State(s) to Queue__jki_lib_state_machine.vi"("State(s) in (\"\")"=w250) -> ("States Out"=w249:string)  [unwired: 14 in]
      }
      frame "Macro: Initialize" {
        w251 = "Data: Initialize\nInitialize Core Data\nUI: Initialize\nUI: Front Panel State >> Open"  # Data: Initialize Initialize Core Data UI: Initialize UI: Front Panel State >> Open
        # "Initialization Macro\n(This is called once, when the VI starts)"
        n88 = call <vilib>:"Add State(s) to Queue__jki_lib_state_machine.vi"("State(s) in Front (\"\")"=w251, "State(s) in (\"\")"=w255) -> ("States Out"=w254:string)  [unwired: 13 in]
      }
      frame "Macro: Exit" {
        # "Exit Macro\n(This is called once, when the VI exits)"
        n89 = Unbundle By Name(w262) -> ("Core.Close Panel on Exit?"=w257:bool)
        n90 = call <vilib>:"Conditional State String__jki_lib_state_machine.vi"("Do State(s)?"=w257, "State"="UI: Front Panel State >> Close") -> ("State Out"=w256:string)  [unwired: 7 in]
        n91 = call <vilib>:"Add State(s) to Queue__jki_lib_state_machine.vi"("State(s) in (\"\")"=w256, "State(s) at Back (\"\")"="UI: Uninitialize\nData: Cleanup\nExit") -> ("States Out"=w260:string)  [unwired: 13 in]
        n92 = call <vilib>:"Add State(s) to Queue__jki_lib_state_machine.vi"("State(s) in Front (\"\")"=w260, "State(s) in (\"\")"=w264) -> ("States Out"=w263:string)  [unwired: 13 in]
      }
      frame "---------- New Category ----------" {
        # "Template Separator\n(You can make a copy of, or modify, this frame)"
        n93 = call <vilib>:"Add State(s) to Queue__jki_lib_state_machine.vi"("State(s) in (\"\")"=w268) -> ("States Out"=w267:string)  [unwired: 14 in]
      }
      frame "New Category: 1" {
        # "Your code here.\n(You can make a copy of, or modify, this frame)"
        n94 = call <vilib>:"Add State(s) to Queue__jki_lib_state_machine.vi"("State(s) in (\"\")"=w272) -> ("States Out"=w271:string)  [unwired: 14 in]
      }
      frame "New Category: 2" {
        # "Your code here.\n(You can make a copy of, or modify, this frame)"
        n95 = call <vilib>:"Add State(s) to Queue__jki_lib_state_machine.vi"("State(s) in (\"\")"=w276) -> ("States Out"=w275:string)  [unwired: 14 in]
      }
      frame "Read camera image" {
        # "path to executable"
        # "make path for the image"
        # "Call the app..."
        # "Read out camera image"
        n96 = Current VI's Path() -> (path=w286:path)
        n97 = Unbundle By Name(w283) -> ("Camera ID"=w289:u8)
        n98 = Build Path(base path=w286, name or relative path="..\\\\..\\\\..\\\\..\\\\artifacts\\\\battery-photo\\\\battery-photo.exe") -> (appended path=w287:path)
        n99 = Build Path(base path=w286, name or relative path="..\\\\temp\\\\sample.jpg") -> (appended path=w284:path)
        n100 = call "Acquire Image.vi"("Camera ID"=w289, "error in (no error)"=w290, "EXE path"=w287, "Save to"=w284) -> ("error out"=w281:errorcluster, "Image path"=w277:path)  [unwired: 6 in]
        n101 = call <vilib>:"Read JPEG File.vi"("error in (no error)"=w281, "path to JPEG file"=w277) -> ("error out"=w278:errorcluster, "image data"=w280:T7)  [unwired: 7 in, 1 out]
        n102 = call <vilib>:"Draw Flattened Pixmap.vi"("image data"=w280) -> ("new picture"=→"Acquired picture":picture)  [unwired: 8 in]
        n103 = Bundle By Name(cluster=w283, "Acquired image"=w277) -> (w282:T5)
      }
      frame "Select image" {
        # "select the image"
        n104 = Unbundle By Name(w293) -> ("Acquired image"=w295:path)
        n105 = Equal?(x="Image selection", y=enum32{"Camera", "File input"}."Camera") -> (x = y?=w297:bool)
        n106 = case shown="False" w297 {
          tunnel: w295 -> [_ w309]
          tunnel: [w301 w309] -> w294
          frame False {
            # "select one from the picture ring"
            n107 = Current VI's Path() -> (path=w306:path)
            n108 = Strip Path(path=w306) -> (stripped path=w305:path)  [unwired: 1 out]
            n109 = Build Path(base path=w305, name or relative path="..\\\\..\\\\..\\\\resources\\\\images") -> (appended path=w303:path)
            n110 = Index Array(array=string[] ["batt_0.jpg"], index="Pict Ring") -> (element=w302:string)
            n111 = Build Path(base path=w303, name or relative path=w302) -> (appended path=w301:path)
          }
          frame True {
            # "just use the same image as acquired"
          }
        }
        n112 = Bundle By Name(cluster=w293, "Acquired image"=w294) -> (w292:T5)
      }
      frame "Execute prompt" {
        w315 = "The image provided should show an AA battery. If the battery is green it is made by JYSK. If the battery is white it is made by Eneloop. If the battery is gray it is made by IKEA. If the battery is light blue it is made by Eneloop. For other colors it is unknown. Read out the voltage and mAh rating. The answer should be a JSON with the following fields: \"Manufacturer\", \"Voltage\", \"Capacity\" and \"Error\". Use error if you have any problems recognizing the data except of manufacturer. The output format example: {\n  \"Manufacturer\": \"JYSK\",\n  \"Voltage\": 1.2,\n  \"Capacity\": 2400,\n  \"Error\": \"\"\n}"  # Prompt text
        # "Run prompt"
        # "get KEY"
        # "get ENV file path"
        n113 = Current VI's Path() -> (path=w319:path)
        n114 = Unbundle By Name(w331) -> ("Acquired image"=w329:path)
        n115 = Strip Path(path=w319) -> (stripped path=w318:path)  [unwired: 1 out]
        n116 = Build Path(base path=w318, name or relative path="gptkeys.env") -> (appended path=w316:path)
        n117 = call "Load Env File.vi"("error in (no error)"=w330, "Env file path"=w316) -> ("error out"=w328:errorcluster, "Variables"=w326:variant)  [unwired: 8 in]
        n118 = Get Variant Attribute(Variant=w326, name="API_KEY", default value (empty Variant)="", error in=w328) -> (value=w323:string, error out=w327:errorcluster)  [unwired: 2 out]
        n119 = call "Run Prompt with IMG.vi"("Prompt text"=w315, "error in (no error)"=w327, "API key"=w323, "path to JPEG file"=w329) -> ("error out"=w321:errorcluster, "body"=w322:string)  [unwired: 6 in]
        n120 = call "Parse out Content.vi"("error in (no error)"=w321, "Response body"=w322) -> ("error out"=w320:errorcluster, "Content"=w311:string)  [unwired: 8 in]
        "Raw content" <- w311
        n121 = Concatenate Strings("Decode content >> ", w311) -> (w310:string)
        n122 = call <vilib>:"Add State(s) to Queue__jki_lib_state_machine.vi"("State(s) in Front (\"\")"=w310, "State(s) in (\"\")"=w313) -> ("States Out"=w314:string)  [unwired: 13 in]
      }
      frame "Decode content" {
        # "Clean up for decoding"
        n123 = call "Clean up JSON.vi"("error in (no error)"=w339, "Content JSON"=w338) -> ("error out"=w337:errorcluster, "Cleaned up JSON"=w336:string)  [unwired: 8 in]
        n124 = Unflatten From JSON(JSON string=w336, type and defaults=T1 {"Manufacturer"="", "Voltage"=0.0, "Capacity"=0, "Error"=""} ("Battery data"), error in (no error)=w337) -> (value=→"Battery data":T1, error out=w333:errorcluster)  [unwired: 4 in]
        "DONE" <- TRUE ("DONE")
      }
    }
  }
  "error out" <- w2
